vi "Clear.vi"(8 "error in (no error)":errorcluster, 11 "Variant DVR in":refnum<data-value>) -> (0 "error out":errorcluster, 3 "Variant DVR out":refnum<data-value>)   [LabVIEW 2019, in "Variant Attributes.lvlib"]
doc: "Clears all attributes in the variant attribute DVR without destroying the value containt in the variant."
uses:
  Variant Attributes.lvlib
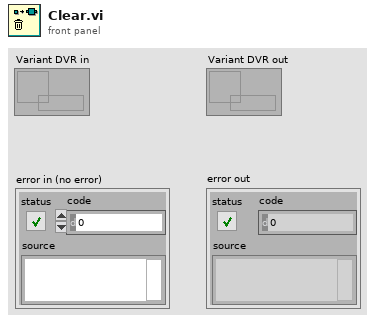
[diagram p1: front panel]
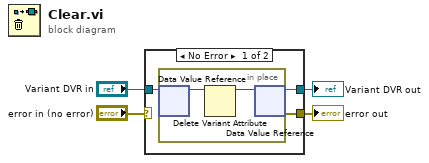
[diagram p0: block diagram]
diagram:
  n1 = case shown="No Error" "error in (no error)" {
    selector: "error in (no error)" -> [_ w10]
    tunnel: "Variant DVR in" -> [w7 w11]
    tunnel: [w6 w11] -> w2
    tunnel: [w5 w10] -> w1
    frame No Error {
      n2 = in-place {
        n3 = in-place-dvr #1(w7) -> (w9:variant)  [unwired: 1 out]
        n4 = Delete Variant Attribute(7:w9) -> (3:w8:variant)  [unwired: 2 in, 2 out]
        n5 = in-place-dvr #1(w8) -> (w6:refnum<data-value>, w5:errorcluster)
      }
    }
    frame Error {
    }
  }
  "error out" <- w1
  "Variant DVR out" <- w2
